vi "随机数-while.vi"() -> ()   [LabVIEW 2012]
panel:
  out "当前的随机数":dbl format="%_10g"
  out "循环次数":i32
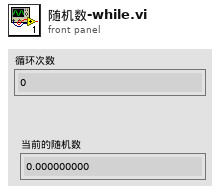
[diagram p1: front panel]
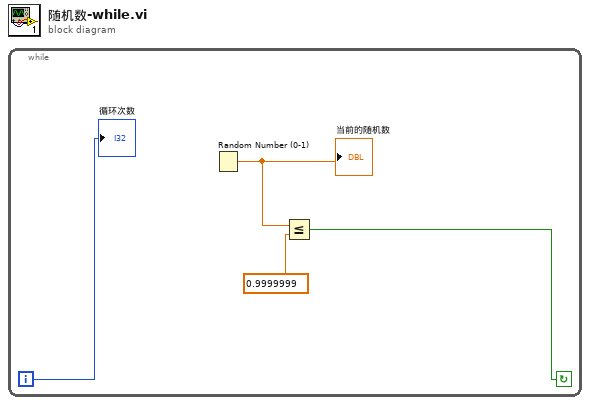
[diagram p0: block diagram]
diagram:
  n1 = while {
    i -> [w4]
    stop <- w1 continue-if-true
    n2 = Random Number (0-1)() -> (number: 0 to 1=w3:dbl)
    "当前的随机数" <- w3
    n3 = Less Or Equal?(x=w3, y=0.9999999) -> (x <= y?=w1:bool)
    "循环次数" <- w4
  }
